vi "Set Server or Cache.vi"(10 "Mode":T1(ring), 11 ".NET Refnum in":refnum<k24>) -> (3 ".NET Refnum out":refnum<k24>)   [LabVIEW 2021, in "NMEA_GPS Ublox M8N.lvlib"]
uses:
  D:/My Projects/Ava Sanjesh Project/VI/GPS uBlox M8N Read/With GMap1.7.0/Data/GMap.NET.WindowsForms.dll
  Data/GMap.NET.WindowsForms.dll
  D:/My Projects/Ava Sanjesh Project/VI/GPS uBlox M8N Read/With GMap1.7.0/Data/GMap.NET.Core.dll
  Data/GMap.NET.Core.dll
  NMEA_GPS Ublox M8N.lvlib
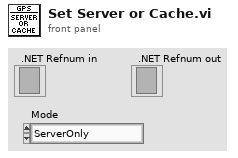
[diagram p1: front panel]
types:
  T1 = enum16{"ServerOnly", "ServerAndCache", "CacheOnly"}
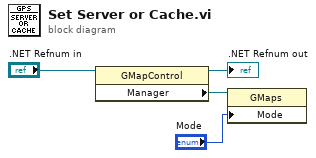
[diagram p0: block diagram]
diagram:
  n1 = property class="GMapControl"(reference=".NET Refnum in") -> (reference out=→".NET Refnum out":refnum<k24>, "Manager"=w2:refnum<k24>)  [unwired: 1 in, 1 out]
  n2 = property class="GMaps"(reference=w2, "Mode"="Mode") -> ()  [unwired: 1 in, 2 out]
